vi "main.vi"() -> ()   [LabVIEW 2017]
uses:
  Baby Human/BabyHuman.lvclass
  C:/dev/LVOOP/OOPintro/Mammal/Mammal.lvclass
  Cat/Cat.lvclass
  Dog/Dog.lvclass
  Human/Human.lvclass
  Mammal/Mammal.lvclass
panel:
  out "class name":string
  out "speak":string
  out "move":string
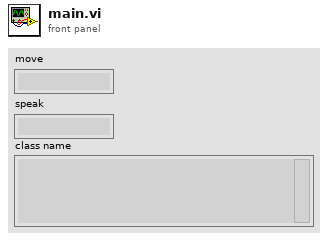
[diagram p1: front panel]
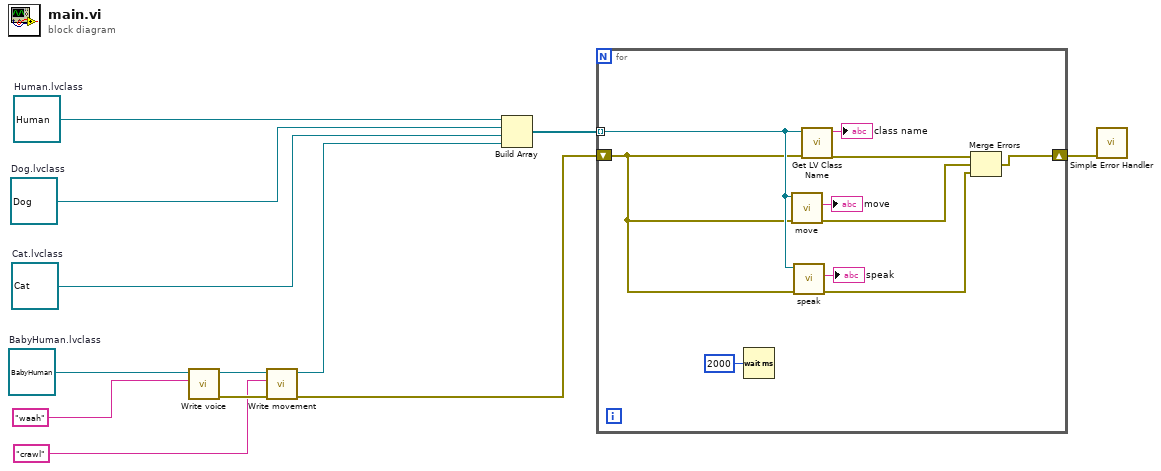
[diagram p0: block diagram]
diagram:
  w7 = refnum<class "Human.lvclass"> refnum  # Human.lvclass
  w6 = refnum<class "Dog.lvclass"> refnum  # Dog.lvclass
  w5 = refnum<class "Cat.lvclass"> refnum  # Cat.lvclass
  w12 = refnum<class "BabyHuman.lvclass"> refnum  # BabyHuman.lvclass
  n1 = call-dynamic "Write voice.vi"("voice"="waah", "BabyHuman in"=w12) -> ("error out"=w9:errorcluster, "BabyHuman out"=w10:refnum<class "BabyHuman.lvclass">)  [unwired: 8 in]
  n2 = call-dynamic "Write movement.vi"("error in (no error)"=w9, "movement"="crawl", "BabyHuman in"=w10) -> ("error out"=w2:errorcluster, "BabyHuman out"=w4:refnum<class "BabyHuman.lvclass">)  [unwired: 7 in]
  n3 = Build Array(w7, w6, w5, w4) -> (w3:refnum<class "Mammal.lvclass">[])
  n4 = for {
    tunnel: w3 -> [w20] mode=indexing
    shift-right: [w14] -> w1
    shift-left: w2 -> [w18]
    n5 = Wait (ms)(milliseconds to wait=u32 2000) -> ()  [unwired: 1 out]
    n6 = call-dynamic "move.vi"("error in (no error)"=w18, "Mammal in"=w20) -> ("error out"=w16:errorcluster, "message"=→"move":string)  [unwired: 7 in, 1 out]
    n7 = call-dynamic "speak.vi"("error in (no error)"=w18, "Mammal in"=w20) -> ("error out"=w15:errorcluster, "message"=→"speak":string)  [unwired: 7 in, 1 out]
    n8 = call <vilib>:"Get LV Class Name.vi"("error in (no error)"=w18, "object"=w20) -> ("error out"=w17:errorcluster, "class name"=→"class name":string)  [unwired: 8 in]
    n9 = Merge Errors(w17, w16, w15) -> (w14:errorcluster)
  }
  n10 = call <vilib>:"Simple Error Handler.vi"("error in (no error)"=w1) -> ()  [unwired: 4 in, 5 out]
